vi "mainFPGA.vi"() -> ()   [LabVIEW 2021]
uses:
  <vilib>/rvi/Emulation/niFpgaGetClockAttributes.vi
  <vilib>/rvi/Emulation/niFpgaSctlEmulationGetInTimedLoop.vi
  <vilib>/rvi/Emulation/niFpgaEmulationReportErrorSimple.vi
  <vilib>/rvi/Emulation/niFpgaCriticalErrorInLSC.vi
panel:
  out "indicatorName2":i16
  in  "controlName2":i16
  out "debugControlRelays":u8
  in  "controlRelays":u8
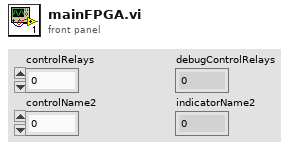
[diagram p1: front panel]
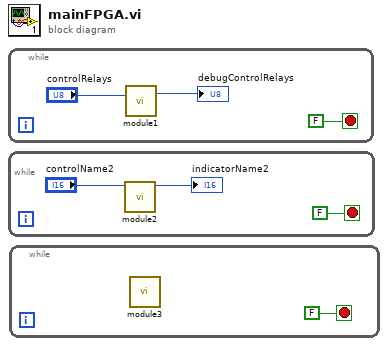
[diagram p0: block diagram]
diagram:
  n1 = while {
    stop <- FALSE stop-if-true
    n2 = call "module1.vi"("controlRelays"="controlRelays") -> ("debugControlRelays"=→"debugControlRelays":u8)  [unwired: 10 in]
  }
  n3 = while {
    stop <- FALSE stop-if-true
    n4 = call "module2.vi"("controlName2"="controlName2") -> ("indicatorName2"=→"indicatorName2":i16)  [unwired: 10 in]
  }
  n5 = while {
    stop <- FALSE stop-if-true
    n6 = call "module3.vi"() -> ()  [unwired: 11 in, 1 out]
  }
